vi "Read or Write Dashboard.vi"   [LabVIEW 2015]
uses:
  Subsystem VIs/Drive SS/Drive Subsystem State.ctl
  <vilib>/Rock Robotics/Network Tables/NT Read Boolean.vi
  Global Variables/Temp Variables.vi
  <vilib>/Rock Robotics/Network Tables/SD Read Boolean.vi
  <vilib>/Rock Robotics/Network Tables/NT Write Boolean.vi
  Global Variables/Sensor Data.vi
  <vilib>/Rock Robotics/Network Tables/NT Write Number.vi
  Global Variables/Vision Processing Data.vi
types:
  T1 = typedef "Drive Subsystem State.ctl" = enum16{"Drive", "Climb", "Auto Target"}
  T2 = cluster{"Distance (ft)":dbl, "Center":cluster{dbl, dbl}, "Normalized Rect":cluster{"Numeric":dbl, "Numeric 2":dbl, "Numeric 3":dbl, "Numeric 5":dbl}}[]
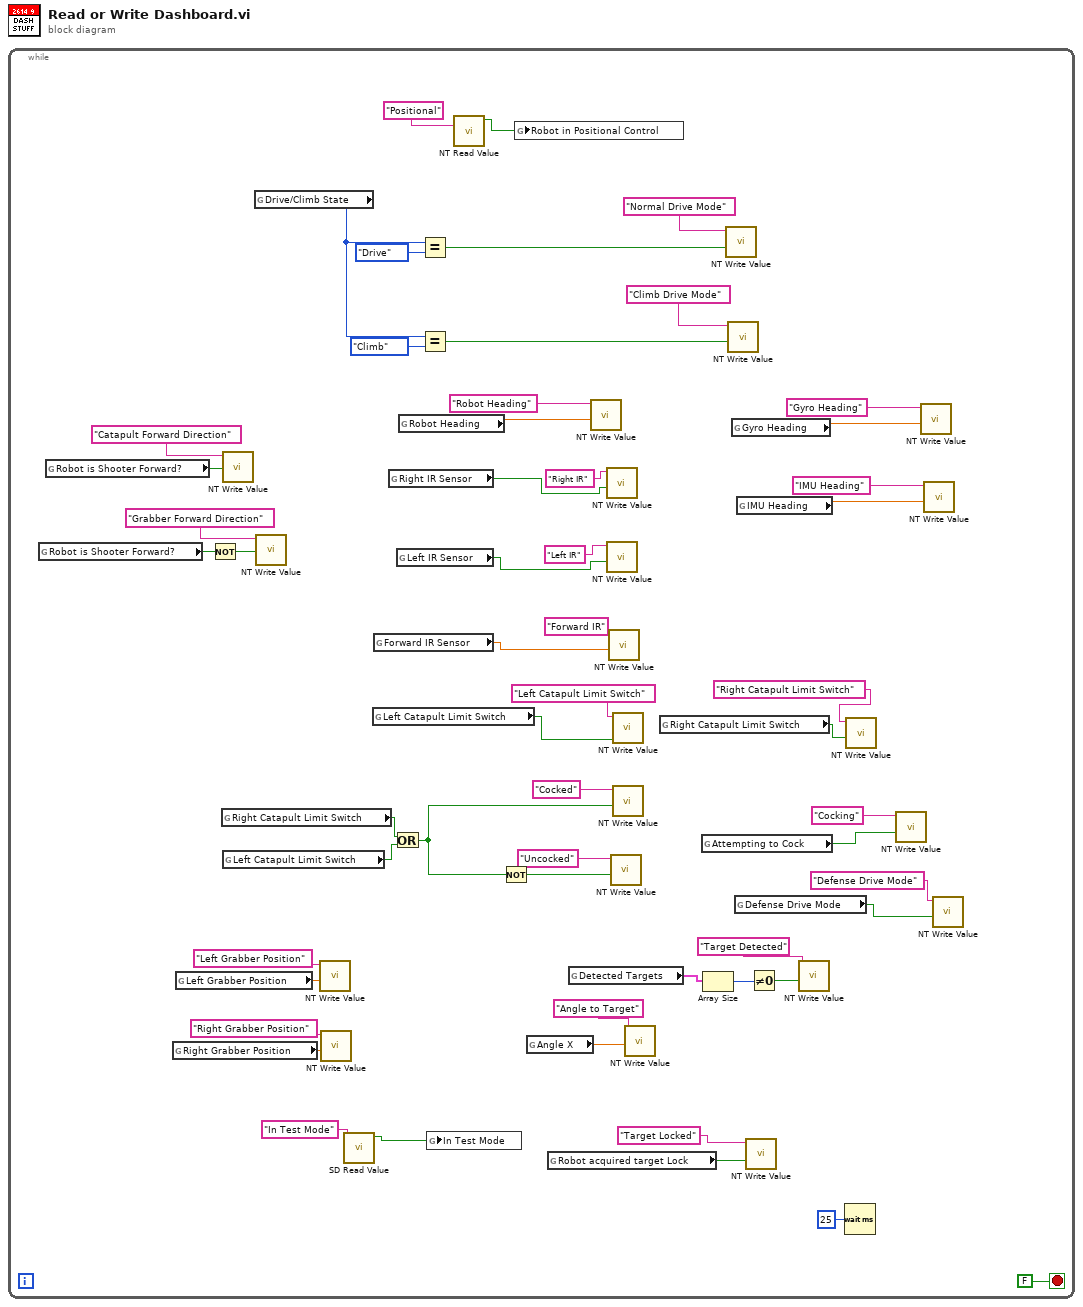
[diagram p0: block diagram]
diagram:
  n1 = while {
    stop <- FALSE stop-if-true
    n2 = global read "Temp Variables.vi" "Robot is Shooter Forward?"() -> (w9:bool)
    n3 = global read "Temp Variables.vi" "Robot is Shooter Forward?"() -> (w10:bool)
    n4 = global read "Sensor Data.vi" "Right Grabber Position"() -> (w29:dbl)
    n5 = global read "Sensor Data.vi" "Left Grabber Position"() -> (w31:dbl)
    n6 = Not(x=w9) -> (.not. x?=w7:bool)
    n7 = global read "Sensor Data.vi" "Right Catapult Limit Switch"() -> (w32:bool)
    n8 = call-poly <vilib>:"NT Write Value.vi"("Boolean"=w10, "Name"="Catapult Forward Direction") -> ()  [unwired: 9 in, 1 out]
    n9 = global read "Sensor Data.vi" "Left Catapult Limit Switch"() -> (w33:bool)
    n10 = global read "Temp Variables.vi" "Drive/Climb State"() -> (w48:T1)
    n11 = call-poly <vilib>:"NT Write Value.vi"("Boolean"=w7, "Name"="Grabber Forward Direction") -> ()  [unwired: 9 in, 1 out]
    n12 = call-poly <vilib>:"NT Write Value.vi"("Numeric"=w31, "Name"="Left Grabber Position") -> ()  [unwired: 9 in, 1 out]
    n13 = call-poly <vilib>:"NT Write Value.vi"("Numeric"=w29, "Name"="Right Grabber Position") -> ()  [unwired: 9 in, 1 out]
    n14 = call-poly <vilib>:"SD Read Value.vi"("Name"="In Test Mode") -> ("Boolean"=w14:bool)  [unwired: 8 in, 2 out]
    n15 = global read "Sensor Data.vi" "Left Catapult Limit Switch"() -> (w38:bool)
    n16 = global read "Sensor Data.vi" "Forward IR Sensor"() -> (w39:dbl)
    n17 = global read "Sensor Data.vi" "Right IR Sensor"() -> (w41:bool)
    n18 = Or(x=w32, y=w33) -> (x .or. y?=w34:bool)
    n19 = global read "Sensor Data.vi" "Left IR Sensor"() -> (w40:bool)
    n20 = global read "Sensor Data.vi" "Robot Heading"() -> (w46:dbl)
    n21 = Equal?(x=w48, y=Drive_Subsystem_State."Drive") -> (x = y?=w52:bool)
    n22 = Equal?(x=w48, y=Drive_Subsystem_State."Climb") -> (x = y?=w50:bool)
    n23 = global write "Temp Variables.vi" "In Test Mode"(w14) -> ()
    n24 = call-poly <vilib>:"NT Read Value.vi"("Name"="Positional") -> ("Boolean"=w55:bool)  [unwired: 9 in, 1 out]
    n25 = Not(x=w34) -> (.not. x?=w35:bool)
    n26 = global write "Temp Variables.vi" "Robot in Positional Control"(w55) -> ()
    n27 = global read "Vision Processing Data.vi" "Angle X"() -> (w27:dbl)
    n28 = global read "Temp Variables.vi" "Robot acquired target Lock"() -> (w5:bool)
    n29 = global read "Vision Processing Data.vi" "Detected Targets"() -> (w24:T2)
    n30 = call-poly <vilib>:"NT Write Value.vi"("Numeric"=w46, "Name"="Robot Heading") -> ()  [unwired: 9 in, 1 out]
    n31 = call-poly <vilib>:"NT Write Value.vi"("Boolean"=w41, "Name"="Right IR") -> ()  [unwired: 9 in, 1 out]
    n32 = call-poly <vilib>:"NT Write Value.vi"("Boolean"=w40, "Name"="Left IR") -> ()  [unwired: 9 in, 1 out]
    n33 = call-poly <vilib>:"NT Write Value.vi"("Numeric"=w39, "Name"="Forward IR") -> ()  [unwired: 9 in, 1 out]
    n34 = call-poly <vilib>:"NT Write Value.vi"("Boolean"=w35, "Name"="Uncocked") -> ()  [unwired: 9 in, 1 out]
    n35 = call-poly <vilib>:"NT Write Value.vi"("Boolean"=w38, "Name"="Left Catapult Limit Switch") -> ()  [unwired: 9 in, 1 out]
    n36 = call-poly <vilib>:"NT Write Value.vi"("Boolean"=w34, "Name"="Cocked") -> ()  [unwired: 9 in, 1 out]
    n37 = call-poly <vilib>:"NT Write Value.vi"("Numeric"=w27, "Name"="Angle to Target") -> ()  [unwired: 9 in, 1 out]
    n38 = global read "Sensor Data.vi" "Right Catapult Limit Switch"() -> (w20:bool)
    n39 = global read "Temp Variables.vi" "Attempting to Cock"() -> (w18:bool)
    n40 = Array Size(array=w24) -> (size(s)=w22:i32)
    n41 = call-poly <vilib>:"NT Write Value.vi"("Boolean"=w52, "Name"="Normal Drive Mode") -> ()  [unwired: 9 in, 1 out]
    n42 = call-poly <vilib>:"NT Write Value.vi"("Boolean"=w50, "Name"="Climb Drive Mode") -> ()  [unwired: 9 in, 1 out]
    n43 = global read "Sensor Data.vi" "Gyro Heading"() -> (w4:dbl)
    n44 = global read "Temp Variables.vi" "Defense Drive Mode"() -> (w13:bool)
    n45 = global read "Sensor Data.vi" "IMU Heading"() -> (w1:dbl)
    n46 = call-poly <vilib>:"NT Write Value.vi"("Boolean"=w5, "Name"="Target Locked") -> ()  [unwired: 9 in, 1 out]
    n47 = Not Equal To 0?(x=w22) -> (x != 0?=w23:bool)
    n48 = call-poly <vilib>:"NT Write Value.vi"("Boolean"=w23, "Name"="Target Detected") -> ()  [unwired: 9 in, 1 out]
    n49 = Wait (ms)(milliseconds to wait=u32 25) -> ()  [unwired: 1 out]
    n50 = call-poly <vilib>:"NT Write Value.vi"("Boolean"=w20, "Name"="Right Catapult Limit Switch") -> ()  [unwired: 9 in, 1 out]
    n51 = call-poly <vilib>:"NT Write Value.vi"("Boolean"=w18, "Name"="Cocking") -> ()  [unwired: 9 in, 1 out]
    n52 = call-poly <vilib>:"NT Write Value.vi"("Numeric"=w4, "Name"="Gyro Heading") -> ()  [unwired: 9 in, 1 out]
    n53 = call-poly <vilib>:"NT Write Value.vi"("Numeric"=w1, "Name"="IMU Heading") -> ()  [unwired: 9 in, 1 out]
    n54 = call-poly <vilib>:"NT Write Value.vi"("Boolean"=w13, "Name"="Defense Drive Mode") -> ()  [unwired: 9 in, 1 out]
  }
